vi "Check Abort.vi"(6 "Loop Data in":T1, 11 "Sequence in":refnum<class "Sequence.lvclass">) -> (4 "Loop Data":T1)   [LabVIEW 2023, in "VolatusSeq.lvlib" / "Sequence.lvclass"]
uses:
  Sequence.lvclass
  Loop Data.ctl
  Volatus/MessageQ/MessageQ.lvclass
  Sequence Time.ctl
  Sequence.lvclass/Sequence.ctl
  State/State.lvclass
  VolatusSeq.lvlib
  VolatusSeqConfig/Debug Flags.ctl
  VolatusSeqConfig/VolatusSeqConfig.lvlib
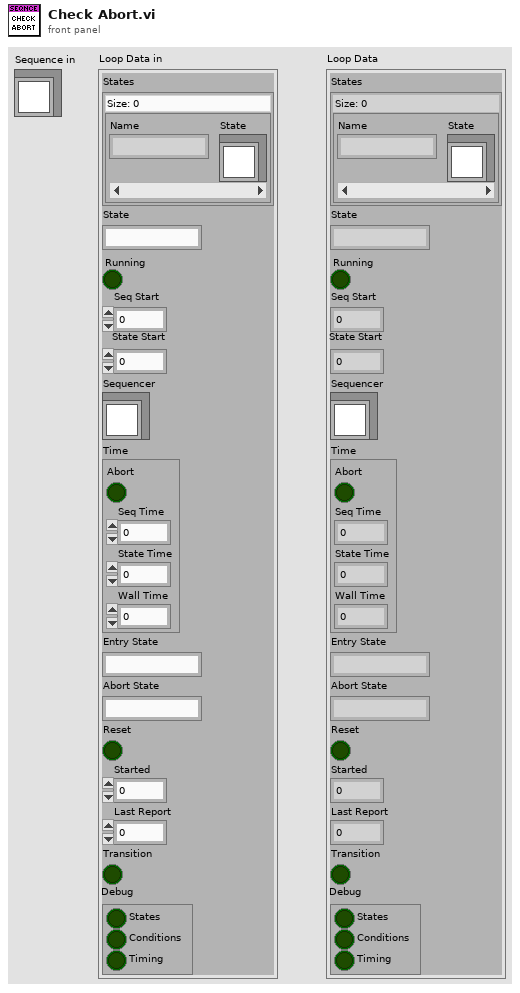
[diagram p1: front panel]
types:
  T1 = typedef "VolatusSeq.lvlib/Sequence.lvclass/Loop Data.ctl" = cluster{"States":map{string, refnum<class "State.lvclass">}, "State":string, "Running":bool, "Seq Start":dbl, "State Start":dbl, "Sequencer":refnum<class "MessageQ.lvclass">, "Time":T2, "Entry State":string, "Abort State":string, "Reset":bool, "Started":dbl, "Last Report":dbl, "Transition":bool, "Debug":T3}
  T2 = typedef "VolatusSeq.lvlib/Sequence Time.ctl" = cluster{"Abort":bool, "Seq Time":dbl, "State Time":dbl, "Wall Time":dbl}
  T3 = typedef "VolatusSeqConfig.lvlib/Debug Flags.ctl" = cluster{"States":bool, "Conditions":bool, "Timing":bool}
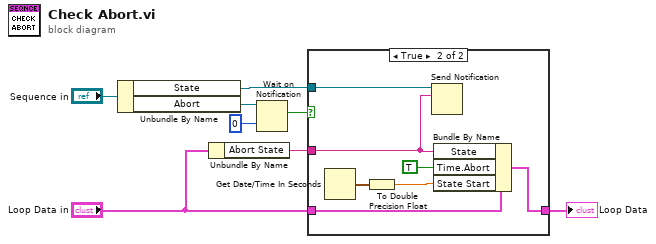
[diagram p0: block diagram]
diagram:
  n1 = Unbundle By Name("Sequence in") -> ("State"=w1:refnum<notifier>, "Abort"=w7:refnum<notifier>)
  n2 = Unbundle By Name("Loop Data in") -> ("Abort State"=w5:string)
  n3 = Wait on Notification(notifier=w7, timeout in ms (-1)=0) -> (notification=w2:bool)  [unwired: 2 in, 3 out]
  n4 = case shown="True" w2 {
    tunnel: w5 -> [_ w13]
    tunnel: "Loop Data in" -> [w9 w12]
    tunnel: [w9 w11] -> w3
    tunnel: w1 -> [_ w10]
    frame False {
    }
    frame True {
      n5 = Get Date/Time In Seconds() -> (seconds since 1Jan1904=w16:timestamp)
      n6 = To Double Precision Float(number=w16) -> (double precision float=w15:dbl)
      n7 = Send Notification(notification=w13, notifier=w10) -> ()  [unwired: 1 in, 2 out]
      n8 = Bundle By Name(cluster=w12, "State"=w13, "Time.Abort"=TRUE ("Abort"), "State Start"=w15) -> (w11:T1)
    }
  }
  "Loop Data" <- w3
